vi "DetectCamerasTest.vi"() -> ()   [LabVIEW 2017]
uses:
  <vilib>/addons/SystemInfoProcess/SystemInfoProcess.lvlib
  <vilib>/addons/InsightCM/Devices/Shared/Utility/DetectCameras/CameraInfo.ctl
panel:
  out "new cameras":T1[](array[typedef])
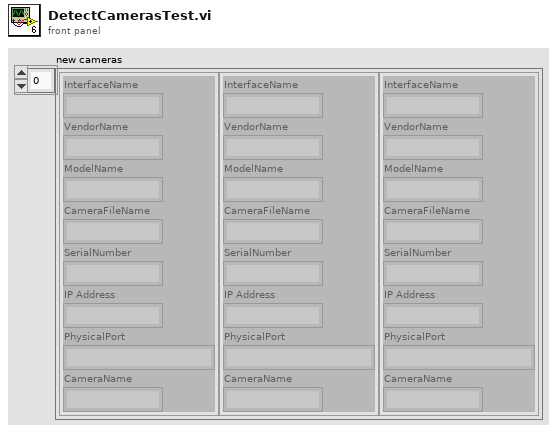
[diagram p1: front panel]
types:
  T1 = typedef "CameraInfo.ctl" = cluster{"InterfaceName":string, "VendorName":string, "ModelName":string, "CameraFileName":string, "SerialNumber":string, "IP Address":string, "PhysicalPort":string, "CameraName":string}
  T2 = typedef "SystemInfoProcess.lvlib/NetworkAdapterSettings.ctl" = cluster{"Adapter Mode":u32, "IsPrimary":bool, "MACAddr":string, "IP Address Request Mode":u32, "IPAddr":string, "SubnetMask":string, "Gateway":string, "DNSServer":string, "Alias":string}
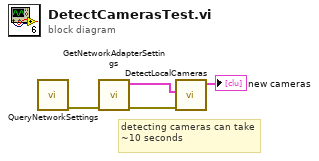
[diagram p0: block diagram]
diagram:
  # "detecting cameras can take ~10 seconds"
  n1 = call <vilib>:"QueryNetworkSettings.vi"() -> ("error out"=w4:errorcluster)  [unwired: 11 in]
  n2 = call <vilib>:"GetNetworkAdapterSettings.vi"("error in (no error)"=w4) -> ("error out"=w3:errorcluster, "Network Adapter Settings"=w2:T2[])  [unwired: 8 in, 1 out]
  n3 = call <vilib>:"DetectLocalCameras.vi"("error in (no error)"=w3, "network configuration"=w2) -> ("new cameras"=→"new cameras":T1[])  [unwired: 8 in, 1 out]
